vi "UpdateUserInterface.vi"(8 "error in (no error)":errorcluster, 10 "DataExchange":T1, 11 "StepMotorController in":refnum<class "StepMotorController.lvclass">) -> (0 "error out":errorcluster, 2 "DataExchange Out":T1, 3 "StepMotorController out":refnum<class "StepMotorController.lvclass">)   [LabVIEW 2020, in "StepMotorController.lvlib" / "StepMotorController.lvclass"]
uses:
  StepMotorController.lvclass
  Model/Hardware Abstraction Layer/Component/Device/Device/DataExchange.ctl
  StepMotorController.lvclass/StepMotorController.ctl
  Model/Hardware Abstraction Layer/Component/GenericActor/GenericActor/GenericController.lvclass
  Interface/DataListener/DataListener.lvclass
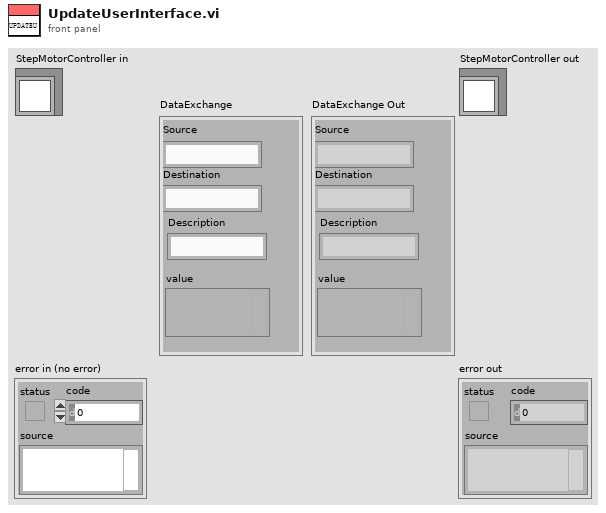
[diagram p1: front panel]
types:
  T1 = typedef "DataListener.lvclass/DataExchange.ctl" = cluster{"Source":string, "Destination":string, "Description":string, "value":variant}
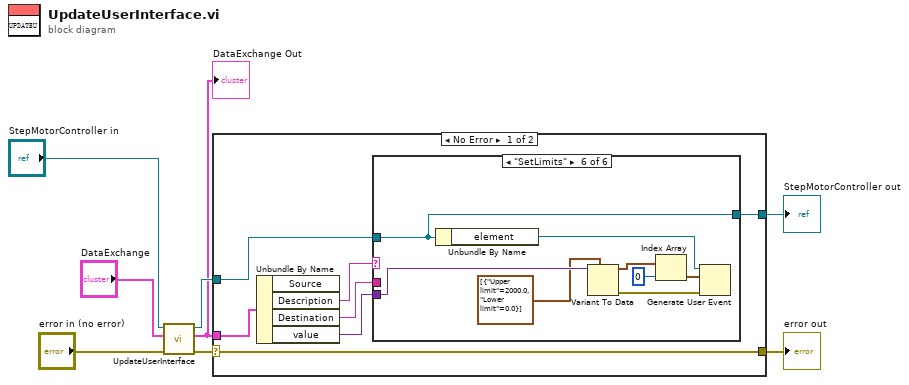
[diagram p0: block diagram]
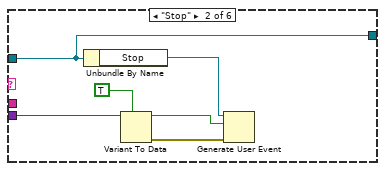
[diagram p3: hidden frame]
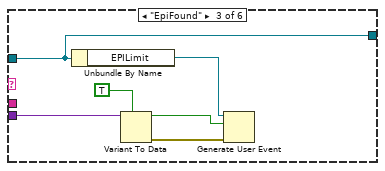
[diagram p4: hidden frame]
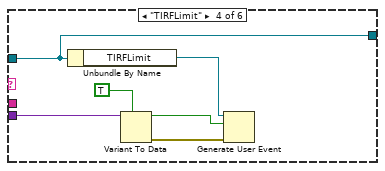
[diagram p5: hidden frame]
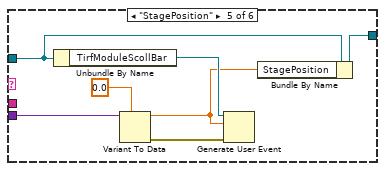
[diagram p6: hidden frame]
diagram:
  n1 = call-parent "UpdateUserInterface.vi"("error in (no error)"="error in (no error)", "DataExchange"="DataExchange", "GenericController in"="StepMotorController in") -> ("error out"=w4:errorcluster, "DataExchange Out"=w1:T1, "GenericController out"=w5:refnum<class "StepMotorController.lvclass">)  [unwired: 6 in]
  "DataExchange Out" <- w1
  n2 = case shown="No Error" w4 {
    selector: w4 -> [w15 w51]
    tunnel: [w15 w51] -> w2
    tunnel: [w9 w50] -> w3
    tunnel: w5 -> [w10 w50]
    tunnel: w1 -> [w14 _]
    frame No Error {
      n3 = Unbundle By Name(w14) -> ("Description"=w11:string, "Destination"=w12:string, "value"=w13:variant)  [unwired: 1 out]
      n4 = case shown="\"SetLimits\"" w11 {
        tunnel: w13 -> [_ w22 w28 w34 w41 w49]
        tunnel: w12 -> [_ _ _ _ _ _]
        tunnel: w10 -> [w16 w17 w23 w29 w37 w42]
        tunnel: [w16 w17 w23 w29 w36 w42] -> w9
        frame Default {
        }
        frame "Stop" {
          n5 = Unbundle By Name(w17) -> ("Stop"=w21:refnum<user-event>)
          n6 = Variant To Data(type=TRUE, Variant=w22) -> (data=w20:bool, error out=w18:errorcluster)  [unwired: 1 in]
          n7 = Generate User Event(user event=w21, event data cluster=w20, error in=w18) -> ()  [unwired: 1 in, 2 out]
        }
        frame "EpiFound" {
          n8 = Unbundle By Name(w23) -> ("EPILimit"=w27:refnum<user-event>)
          n9 = Variant To Data(type=TRUE, Variant=w28) -> (data=w26:bool, error out=w24:errorcluster)  [unwired: 1 in]
          n10 = Generate User Event(user event=w27, event data cluster=w26, error in=w24) -> ()  [unwired: 1 in, 2 out]
        }
        frame "TIRFLimit" {
          n11 = Unbundle By Name(w29) -> ("TIRFLimit"=w33:refnum<user-event>)
          n12 = Variant To Data(type=TRUE, Variant=w34) -> (data=w32:bool, error out=w30:errorcluster)  [unwired: 1 in]
          n13 = Generate User Event(user event=w33, event data cluster=w32, error in=w30) -> ()  [unwired: 1 in, 2 out]
        }
        frame "StagePosition" {
          n14 = Unbundle By Name(w37) -> ("TirfModuleScollBar"=w40:refnum<user-event>)
          n15 = Variant To Data(type=0.0 ("event data"), Variant=w41) -> (data=w35:dbl, error out=w39:errorcluster)  [unwired: 1 in]
          n16 = Generate User Event(user event=w40, event data cluster=w35, error in=w39) -> ()  [unwired: 1 in, 2 out]
          n17 = Bundle By Name(cluster=w37, "StagePosition"=w35) -> (w36:refnum<class "StepMotorController.lvclass">)
        }
        frame "SetLimits" {
          n18 = Unbundle By Name(w42) -> ("element"=w48:refnum<user-event>)
          n19 = Variant To Data(type=cluster{"Upper limit":dbl, "Lower limit":dbl}[] [{"Upper limit"=2000.0, "Lower limit"=0.0}] ("Limits"), Variant=w49) -> (data=w45:cluster{"Upper limit":dbl, "Lower limit":dbl}[], error out=w47:errorcluster)  [unwired: 1 in]
          n20 = Index Array(array=w45, index=0) -> (element=w43:cluster{"Upper limit":dbl, "Lower limit":dbl})
          n21 = Generate User Event(user event=w48, event data cluster=w43, error in=w47) -> ()  [unwired: 1 in, 2 out]
        }
      }
    }
    frame Error {
    }
  }
  "error out" <- w2
  "StepMotorController out" <- w3
